vi "ASM.Reset.vi"(8 "error in (no error)":errorcluster, 11 "ActorStateMachine in":refnum<class "ActorStateMachine.lvclass">) -> (0 "error out":errorcluster, 3 "ActorStateMachine out":refnum<class "ActorStateMachine.lvclass">)   [LabVIEW 2021, in "ActorStateMachine.lvlib" / "ActorStateMachine.lvclass"]
uses:
  ActorStateMachine.lvclass
  ActorStateMachine.lvclass/ActorStateMachine.ctl
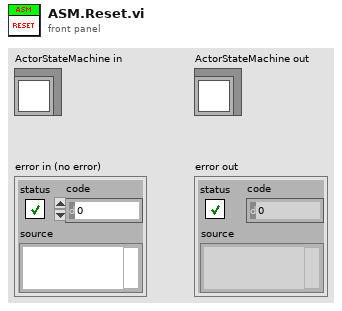
[diagram p1: front panel]
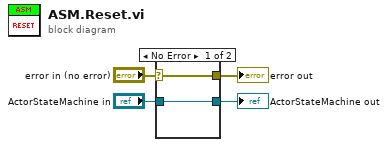
[diagram p0: block diagram]
diagram:
  n1 = case shown="No Error" "error in (no error)" {
    selector: "error in (no error)" -> [w6 w8]
    tunnel: [w6 w8] -> w3
    tunnel: [w5 w7] -> w1
    tunnel: "ActorStateMachine in" -> [w5 w7]
    frame No Error {
    }
    frame Error {
    }
  }
  "error out" <- w3
  "ActorStateMachine out" <- w1
